vi "Periodic Tasks.vi"(8 "error in (no error)":errorcluster) -> ()   [LabVIEW 2016]
doc: "This VI runs in parallel to other tasks. It can contain as many user-defined periodic loops as you need. These can carry out PID or other sorts of timed response."
uses:
  <vilib>/Rock Robotics/WPI/DriverStation/WPI_DriverStationRobotMode2.ctl
  Robot Global Data.vi
  <vilib>/Rock Robotics/Network Tables/NT Read String.vi
  <vilib>/Rock Robotics/Network Tables/NT Read Number.vi
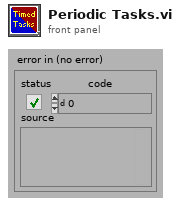
[diagram p1: front panel]
types:
  T1 = cluster{"theta":dbl, "distance":dbl, "x":dbl, "y":dbl}[]
  T2 = typedef "WPI_EncoderDevRef.ctl" = cluster{"DevStatus":errorcluster, "EncoderIndex":T3, "CounterIndex":T4, "DistancePerCount":dbl, "Decoding Type":T5}
  T3 = typedef "FPGA_EncoderIdx.ctl" = enum8{"Enc 0", "Enc 1", "Enc 2", "Enc 3", "Enc 4", "Enc 5", "Enc 6", "Enc 7", "Invalid"}
  T4 = typedef "FPGA_CounterCtrSystemIndex.ctl" = enum8{"Ctr 0", "Ctr 1", "Ctr 2", "Ctr 3", "Ctr 4", "Ctr 5", "Ctr 6", "Ctr 7", "Invalid"}
  T5 = typedef "WPI_EncoderType.ctl" = enum16{"1x", "2x", "4x"}
  T6 = typedef "WPI_RobotDriveDevRef.ctl" = cluster{"DevStatus":errorcluster, "Motors[]":T7[], "Square Inputs":bool, "Max Output":dbl}
  T7 = typedef "WPI_MotorControlDeviceRef.ctl" = cluster{"DeviceStatus":errorcluster, "Type":T8, "PWM":cluster{"PWM Channel":T9, "DeadBand":T10}, "CAN":cluster{"Device Number":u8, "SetOutput VI Ref":variant, "GetOutput VI Ref":variant, "Enable VI Ref":variant, "Disable VI Ref":variant, "Data":variant}, "Invert":bool}
  T8 = typedef "WPI_MotorControlType.ctl" = enum16{"PWM", "CAN"}
  T9 = typedef "FPGA_DIOPWMChannel.ctl" = enum8{"PWM 0", "PWM 1", "PWM 2", "PWM 3", "PWM 4", "PWM 5", "PWM 6", "PWM 7", "PWM 8", "PWM 9", "PWM MXP 0", "PWM MXP 1", "PWM MXP 2", "PWM MXP 3", "PWM MXP 4", "PWM MXP 5", "PWM MXP 6", "PWM MXP 7", "PWM MXP 8", "PWM MXP 9", "Invalid"}
  T10 = typedef "WPI_PWMDeadband.ctl" = cluster{"Name":string, "maxPositivePwm":i32, "minPositivePwm":i32, "centerPwm":i32, "maxNegativePwm":i32, "minNegativePwm":i32, "angularRange":u16}
  T11 = cluster{"theta":dbl, "distance":dbl, "x":dbl, "y":dbl}
  T12 = cluster{"Yaw":dbl, "Roll":dbl, "Pitch":dbl, "Heading":dbl, "Fused Heading":dbl}
  T13 = cluster{"Angle Out":dbl, "Angle Out":dbl, dbl, dbl}
  T14 = typedef "WPI_DriverStationRobotMode2.ctl" = enum16{"Autonomous Disabled", "Autonomous Enabled", "Teleop Disabled", "Teleop Enabled", "Disconnected", "Finish", "Test Disabled", "Test Enabled", "Emergency Stopped"}
  T15 = typedef "WPI_SolenoidDevRef.ctl" = cluster{"DevStatus":errorcluster, "Pneumatics Control Module":u8, "Forward Solenoid Channel":T16, "Reverse Solenoid Channel":T16}
  T16 = typedef "WPI_SolenoidChannel.ctl" = enum8{"Solenoid 0", "Solenoid 1", "Solenoid 2", "Solenoid 3", "Solenoid 4", "Solenoid 5", "Solenoid 6", "Solenoid 7", "Invalid"}
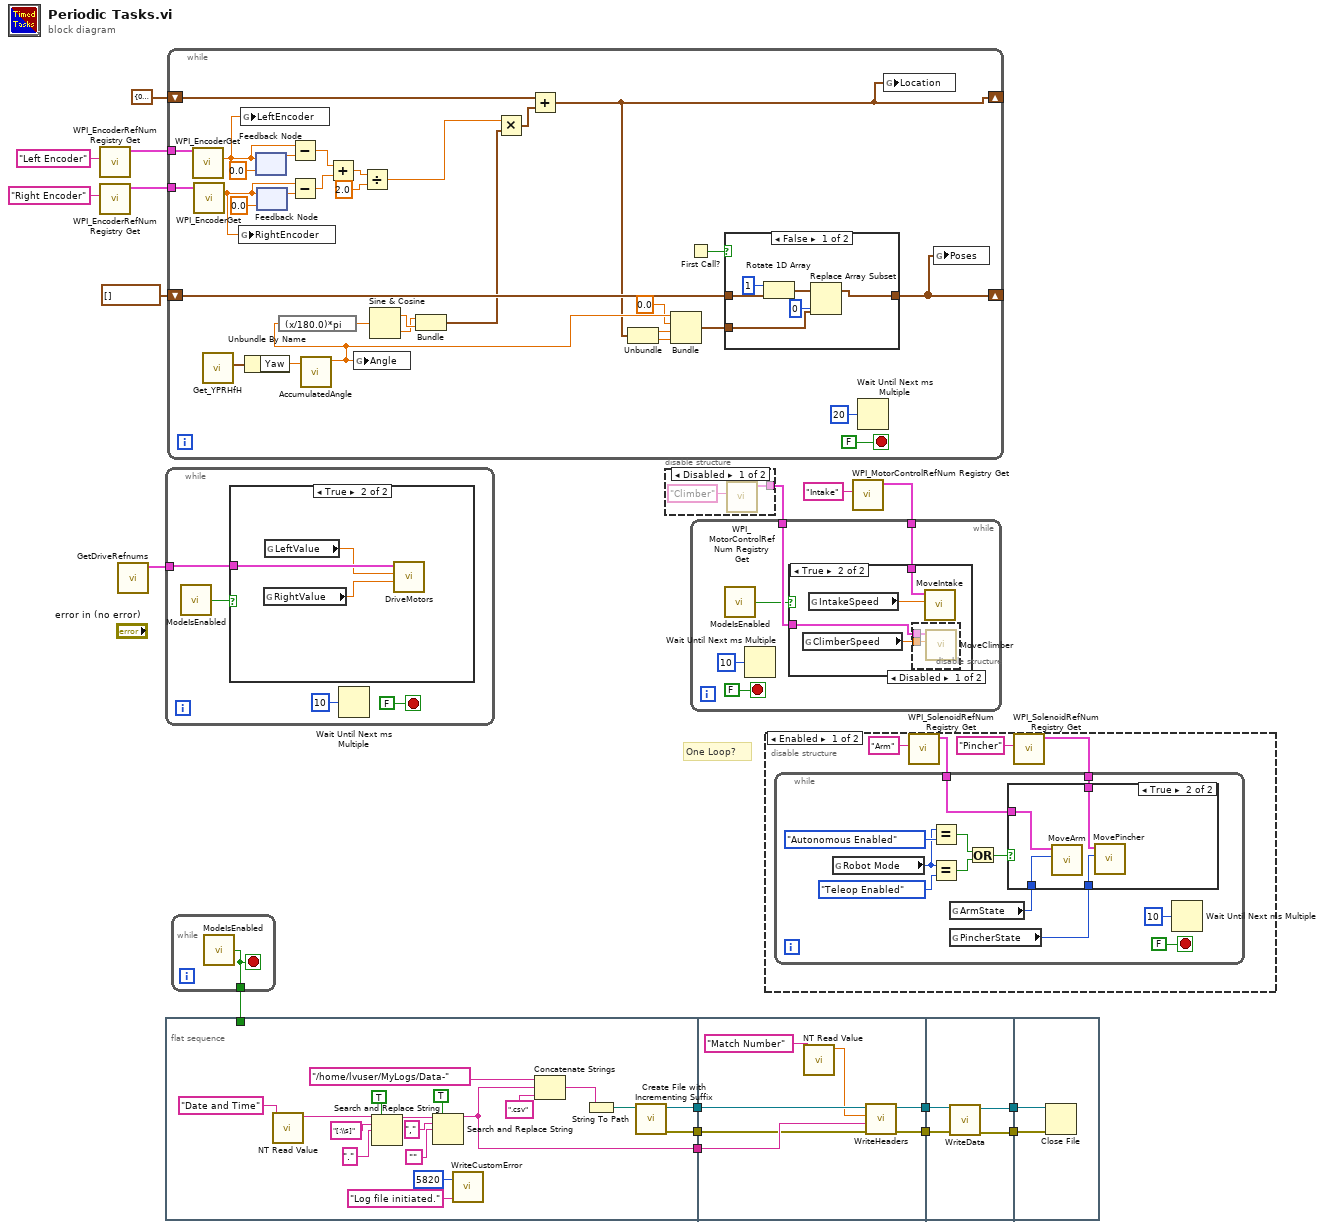
[diagram p0: block diagram]
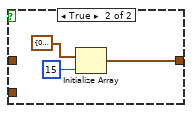
[diagram p7: hidden frame]
diagram:
  # "One Loop?"
  n1 = call <vilib>:"WPI_EncoderRefNum Registry Get.vi"("refnum name"="Left Encoder") -> ("EncoderDevRef"=w5:T2)  [unwired: 9 in, 1 out]
  n2 = call <vilib>:"WPI_EncoderRefNum Registry Get.vi"("refnum name"="Right Encoder") -> ("EncoderDevRef"=w6:T2)  [unwired: 9 in, 1 out]
  n3 = call "GetDriveRefnums.vi"() -> ("Refnums"=w18:T6[])  [unwired: 11 in]
  n4 = while {
    tunnel: w18 -> [w21]
    stop <- FALSE stop-if-true
    n5 = call "ModeIsEnabled.vi"() -> ("enabled?"=w19:bool)  [unwired: 1 in]
    n6 = case shown="True" w19 {
      tunnel: w21 -> [_ w25]
      frame False {
      }
      frame True {
        n7 = global read "Robot Global Data.vi" "RightValue"() -> (w23:dbl)
        n8 = global read "Robot Global Data.vi" "LeftValue"() -> (w24:dbl)
        n9 = call "DriveMotors.vi"("Right"=w23, "Left"=w24, "Refnums"=w25) -> ()  [unwired: 8 in, 1 out]
      }
    }
    n10 = Wait Until Next ms Multiple(millisecond multiple=u32 10) -> ()  [unwired: 1 out]
  }
  n11 = flat-sequence {
    tunnel: [w38] -> w17
    tunnel: [w28] -> w16
    tunnel: [w37] -> w15
    tunnel: w14 -> [_]
    tunnel: w17 -> [w49]
    tunnel: w16 -> [w47]
    tunnel: w15 -> [w46]
    tunnel: [w45] -> w13
    tunnel: [w44] -> w11
    tunnel: w13 -> [w54]
    tunnel: [w51] -> w12
    tunnel: w11 -> [w53]
    tunnel: [w52] -> w10
    tunnel: w12 -> [w56]
    tunnel: w10 -> [w55]
    frame #0 {
      n12 = call-poly <vilib>:"NT Read Value.vi"("Name"="Date and Time") -> ("String"=w29:string)  [unwired: 9 in, 1 out]
      n13 = Search and Replace String(replace all?=TRUE ("replace all? (F)"), input string=w29, search string="[:\\s]", replace string="." ("replace string (\"\")")) -> (result string=w33:string)  [unwired: 4 in, 3 out]
      n14 = Search and Replace String(replace all?=TRUE ("replace all? (F)"), input string=w33, search string=",", replace string="") -> (result string=w28:string)  [unwired: 4 in, 3 out]
      n15 = call "WriteCustomError.vi"("Source"="Log file initiated.", "Code"=u32 5820) -> ()  [unwired: 1 out]
      n16 = Concatenate Strings("/home/lvuser/MyLogs/Data-" ("string"), w28, ".csv" ("string")) -> (w40:string)
      n17 = String To Path(string=w40) -> (path=w39:path)
      n18 = call <vilib>:"Create File with Incrementing Suffix.vi"("file path"=w39) -> ("error out"=w37:errorcluster, "refnum out"=w38:refnum<file>)  [unwired: 8 in, 1 out]
    }
    frame #1 {
      n19 = call-poly <vilib>:"NT Read Value.vi"("Name"="Match Number") -> ("Numeric"=w48:dbl)  [unwired: 9 in, 1 out]
      n20 = call "WriteHeaders.vi"("error in"=w46, "Date and Time"=w47, "Match Number"=w48, "refnum in"=w49) -> ("error out"=w44:errorcluster, "refnum out"=w45:refnum<file>)  [unwired: 6 in]
    }
    frame #2 {
      n21 = call "WriteData.vi"("error in"=w53, "refnum in"=w54) -> ("error out"=w52:errorcluster, "refnum out"=w51:refnum<file>)  [unwired: 8 in]
    }
    frame #3 {
      n22 = Close File(refnum=w56, error in=w55) -> ()  [unwired: 2 out]
    }
  }
  n23 = while {
    shift-right: [w85] -> _
    shift-left: T1 [] ("Poses") -> [w84]
    tunnel: w6 -> [w80]
    tunnel: w5 -> [w79]
    shift-right: [w60] -> _
    shift-left: cluster{"x":dbl, "y":dbl} {"x"=0.0, "y"=0.0} ("Location") -> [w64]
    stop <- FALSE stop-if-true
    n24 = call <vilib>:"WPI_EncoderGet.vi"("EncoderDevRef"=w79) -> ("Distance"=w58:dbl)  [unwired: 5 in, 5 out]
    n25 = call <vilib>:"WPI_EncoderGet.vi"("EncoderDevRef"=w80) -> ("Distance"=w57:dbl)  [unwired: 5 in, 5 out]
    n26 = call <vilib>:"Get_YPRHfH.vi"() -> ("YRPHfH"=w83:T12)  [unwired: 11 in]
    n27 = global write "Robot Global Data.vi" "RightEncoder"(w57) -> ()
    n28 = global write "Robot Global Data.vi" "LeftEncoder"(w58) -> ()
    n29 = Unbundle By Name(w83) -> ("Yaw"=w82:dbl)
    n30 = feedback-in #1(w58) -> ()
    n31 = feedback #1(0.0 ("Distance")) -> (w76:dbl)
    n32 = feedback #2(0.0 ("Distance")) -> (w75:dbl)
    n33 = feedback-in #2(w57) -> ()
    n34 = Subtract(x=w58, y=w76) -> (x-y=w74:dbl)
    n35 = Subtract(x=w57, y=w75) -> (x-y=w73:dbl)
    n36 = call "AccumulatedAngle.vi"("Angle In"=w82) -> ("Angle Out"=w63:dbl)  [unwired: 10 in]
    n37 = expression code="(x/180.0)*pi" ("degrees to radians")(w63) -> (w70:dbl)
    n38 = Add(x=w74, y=w73) -> (x+y=w72:dbl)
    n39 = global write "Robot Global Data.vi" "Angle"(w63) -> ()
    n40 = Divide(x=w72, y=2.0) -> (x/y=w66:dbl)
    n41 = Sine & Cosine(0:w70) -> (1:w69:dbl, 2:w68:dbl)
    n42 = Bundle(w68, w69) -> (w67:cluster{dbl, dbl})  [unwired: 1 in]
    n43 = Multiply(x=w66, y=w67) -> (x*y=w65:cluster{dbl, dbl})
    n44 = Add(x=w64, y=w65) -> (x+y=w60:cluster{dbl, dbl})
    n45 = Unbundle(w60) -> (w62:dbl, w61:dbl)
    n46 = Bundle("Angle Out"=w63, "Angle Out"=0.0, w62, w61) -> (w81:T13)  [unwired: 1 in]
    n47 = First Call?() -> (First Call?: T/F=w86:bool)
    n48 = case shown="False" w86 {
      tunnel: [w91 w95] -> w85
      tunnel: w84 -> [w94 _]
      tunnel: w81 -> [w89 _]
      frame False {
        n49 = Rotate 1D Array(1:w94, 2:1 ("n")) -> (0:w92:T1)
        n50 = Replace Array Subset(array=w92, new element=w89, index=0) -> (w91:T1)
      }
      frame True {
        n51 = Initialize Array(T11 {"theta"=0.0, "distance"=0.0, "x"=0.0, "y"=0.0} ("Poses"), 15 ("dimension size")) -> (w95:T1)
      }
    }
    n52 = Wait Until Next ms Multiple(millisecond multiple=u32 20) -> ()  [unwired: 1 out]
    n53 = global write "Robot Global Data.vi" "Location"(w60) -> ()
    n54 = global write "Robot Global Data.vi" "Poses"(w85) -> ()
  }
  n55 = while {
    tunnel: [w98] -> w14
    stop <- w98 stop-if-true
    n56 = call "ModeIsEnabled.vi"() -> ("enabled?"=w98:bool)  [unwired: 1 in]
  }
  n57 = disable-structure shown="Disabled" {
    disable-tunnel: [w99 _] -> w1
    frame Disabled {
      n58 = call <vilib>:"WPI_MotorControlRefNum Registry Get.vi"("refnum name"="Climber") -> ("MotorControlDevRef"=w99:T7)  [unwired: 9 in, 1 out]
    }
    frame Enabled {
    }
  }
  n59 = disable-structure shown="Enabled" {
    frame Enabled {
      n60 = call <vilib>:"WPI_SolenoidRefNum Registry Get.vi"("refnum name"="Arm") -> ("SolenoidDevRef"=w101:T15)  [unwired: 9 in, 1 out]
      n61 = call <vilib>:"WPI_SolenoidRefNum Registry Get.vi"("refnum name"="Pincher") -> ("SolenoidDevRef"=w102:T15)  [unwired: 9 in, 1 out]
      n62 = while {
        tunnel: w102 -> [w106]
        tunnel: w101 -> [w105]
        stop <- FALSE stop-if-true
        n63 = global read "Robot Global Data.vi" "Robot Mode"() -> (w114:T14)
        n64 = Equal?(x=w114, y=WPI_DriverStationRobotMode2."Autonomous Enabled") -> (x = y?=w112:bool)
        n65 = Equal?(x=w114, y=WPI_DriverStationRobotMode2."Teleop Enabled") -> (x = y?=w111:bool)
        n66 = global read "Robot Global Data.vi" "ArmState"() -> (w108:enum16{"Up", "Down"})
        n67 = global read "Robot Global Data.vi" "PincherState"() -> (w107:enum16{"Open", "Close"})
        n68 = Or(x=w112, y=w111) -> (x .or. y?=w110:bool)
        n69 = case shown="True" w110 {
          tunnel: w108 -> [_ w120]
          tunnel: w107 -> [_ w119]
          tunnel: w106 -> [_ w118]
          tunnel: w105 -> [_ w117]
          frame False {
          }
          frame True {
            n70 = call "MoveArm.vi"("ArmState"=w120, "SolenoidDevRef"=w117) -> ()  [unwired: 10 in]
            n71 = call "MovePincher.vi"("PincherState"=w119, "SolenoidDevRef"=w118) -> ()  [unwired: 10 in]
          }
        }
        n72 = Wait Until Next ms Multiple(millisecond multiple=u32 10) -> ()  [unwired: 1 out]
      }
    }
    frame Disabled {
    }
  }
  n73 = call <vilib>:"WPI_MotorControlRefNum Registry Get.vi"("refnum name"="Intake") -> ("MotorControlDevRef"=w2:T7)  [unwired: 9 in, 1 out]
  n74 = while {
    tunnel: w2 -> [w123]
    tunnel: w1 -> [w122]
    stop <- FALSE stop-if-true
    n75 = call "ModeIsEnabled.vi"() -> ("enabled?"=w121:bool)  [unwired: 1 in]
    n76 = Wait Until Next ms Multiple(millisecond multiple=u32 10) -> ()  [unwired: 1 out]
    n77 = case shown="True" w121 {
      tunnel: w123 -> [_ w128]
      tunnel: w122 -> [_ w126]
      frame False {
      }
      frame True {
        n78 = global read "Robot Global Data.vi" "ClimberSpeed"() -> (w127:dbl)
        n79 = global read "Robot Global Data.vi" "IntakeSpeed"() -> (w129:dbl)
        n80 = disable-structure shown="Disabled" {
          disable-tunnel: w127 -> [w131 _]
          disable-tunnel: w126 -> [w130 _]
          frame Disabled {
            n81 = call "MoveClimber.vi"("Speed"=w131, "MotorControlDevRef"=w130) -> ()  [unwired: 10 in]
          }
          frame Enabled {
          }
        }
        n82 = call "MoveIntake.vi"("Speed"=w129, "MotorControlDevRef"=w128) -> ()  [unwired: 10 in]
      }
    }
  }
